vi "Formatted Timestamp.vi"(11 "Timestamp (now)":timestamp) -> (3 "String Formatted timestamp":string)   [LabVIEW 2017]
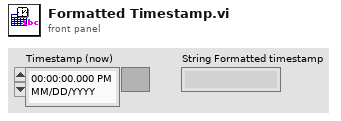
[diagram p1: front panel]
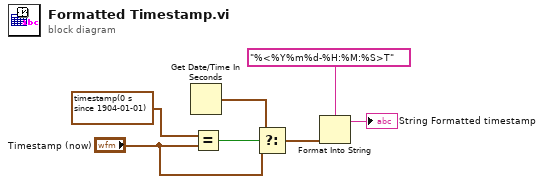
[diagram p0: block diagram]
diagram:
  n1 = Get Date/Time In Seconds() -> (seconds since 1Jan1904=w1:timestamp)
  n2 = Equal?(x=timestamp(0 s since 1904-01-01) ("y"), y="Timestamp (now)") -> (x = y?=w4:bool)
  n3 = Select(t=w1, s=w4, f="Timestamp (now)") -> (s? t:f=w2:timestamp)
  n4 = Format Into String(format string="%<%Y%m%d-%H:%M:%S>T", w2) -> (resulting string=→"String Formatted timestamp":string)  [unwired: 2 in, 1 out]
